vi "Receive Control Mouse Up Event.vi"(8 "error in (no error)":errorcluster, 10 "ControlMouseUpMsg":refnum<class "ControlMouseUpMsg.lvclass">, 11 "GarphView In":refnum<class "GarphView.lvclass">) -> (0 "error out":errorcluster, 3 "GarphView Out":refnum<class "GarphView.lvclass">)   [LabVIEW 2020, in "GarphView.lvlib" / "GarphView.lvclass"]
doc: "<License>\nCopyright © 2017 Composed Systems, LLC | All rights reserved\nwww.composed.io\n\nAuthor: Ethan Stern <ethan.stern@composed.io>\n\nThis software is provided \"AS IS\" WITHOUT WARRANTIES, either express or implied, AND IS FOR EDUCATIONAL PURPOSES ONLY.\n</License>"
uses:
  <vilib>/gpm_packages/@cs/mva-viewable/Source/ActorEvents/IEventAggregator Messages/ControlMouseUpMsg/ControlMouseUpMsg.lvclass
  GarphView.lvclass
  GarphView.lvclass/GarphView.ctl
  <vilib>/gpm_packages/@cs/mva-viewable/Source/IViewable/IViewable/IViewable.lvclass
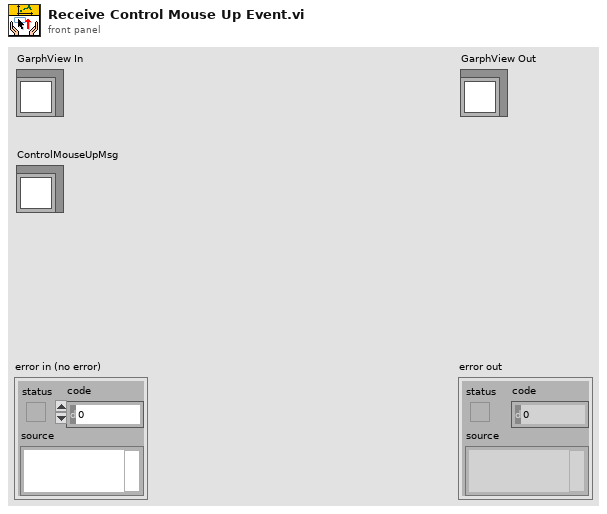
[diagram p1: front panel]
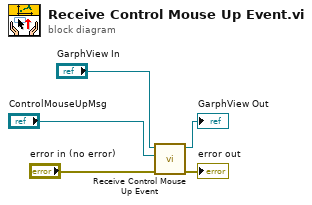
[diagram p0: block diagram]
diagram:
  n1 = call-parent "Receive Control Mouse Up Event.vi"("error in (no error)"="error in (no error)", "ControlMouseUpMsg"="ControlMouseUpMsg", "IEventAggregator In"="GarphView In") -> ("error out"=→"error out":errorcluster, "IEventAggregator Out"=→"GarphView Out":refnum<class "GarphView.lvclass">)  [unwired: 7 in]
